vi "Iniciar.vi"() -> ()   [LabVIEW 2015]
uses:
  <vilib>/addons/_office/excel.llb/Excel Get Data (i32).vi
  <vilib>/Utility/NIReport.llb/NI_report.lvclass
  <vilib>/Utility/NIReport.llb/Excel/NI_Excel.lvclass
  <vilib>/addons/_office/NI_ReportGenerationToolkit.lvlib
panel:
  out "Init Data Out":u16[](array[numeric])
  out "Sheet 3 Data":i32
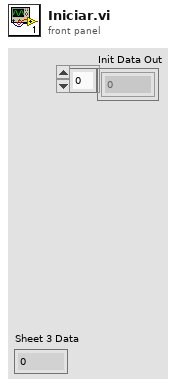
[diagram p1: front panel]
types:
  T1 = enum16{"Standard Report", "HTML", "Word", "Excel"}
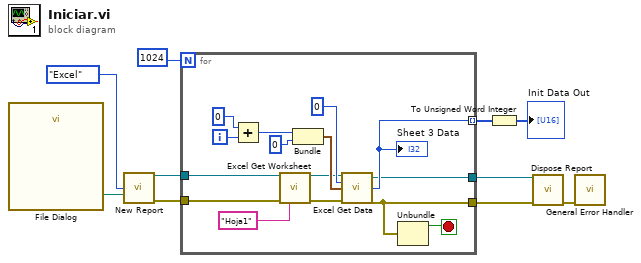
[diagram p0: block diagram]
diagram:
  n1 = call "File Dialog"() -> ("selected path"=w7:path)  [unwired: 7 in, 8 out]
  n2 = call <vilib>:"New Report.vi"("report type"=T1."Excel", "template (empty)"=w7) -> ("report out"=w5:refnum<class "NI_report.lvclass">, "error out"=w4:errorcluster)  [unwired: 4 in, 8 out]
  n3 = for {
    N: 1024 -> [_]
    tunnel: [w16] -> w9 mode=indexing
    tunnel: w5 -> [w15]
    tunnel: w4 -> [w14]
    tunnel: [w13] -> w2
    tunnel: [w12] -> w1
    i -> [w19]
    stop <- w11 stop-if-true
    n4 = Add(x=0, y=w19) -> (x+y=w17:i32)
    n5 = call <vilib>:"Excel Get Worksheet.vi"("report in"=w15, "error in (no error)"=w14, "name (\"\")"="Hoja1" ("name (\"\")")) -> ("report out"=w22:refnum<class "NI_report.lvclass">, "error out"=w21:errorcluster)  [unwired: 1 in, 10 out]
    n6 = Bundle(w17, "worksheet index (0)"=0) -> (w25:cluster{i32, "worksheet index (0)":i32})  [unwired: 1 in]
    n7 = call-poly <vilib>:"Excel Get Data.vi"("report in"=w22, "data type"=0, "start (0, 0)"=w25, "error in (no error)"=w21) -> ("report out"=w13:refnum<class "NI_report.lvclass">, "data"=w16:i32, "error out"=w12:errorcluster)  [unwired: 9 out]
    "Sheet 3 Data" <- w16
    n8 = Unbundle(w12) -> ("status"=w11:bool)  [unwired: 2 out]
  }
  n9 = To Unsigned Word Integer(number=w9) -> (unsigned 16bit integer=→"Init Data Out":u16[])
  n10 = call-dynamic "Dispose Report.vi"("report in"=w2, "error in (no error)"=w1) -> ("error out"=w3:errorcluster)  [unwired: 3 in, 10 out]
  n11 = call <vilib>:"General Error Handler.vi"("error in (no error)"=w3) -> ()  [unwired: 3 in, 12 out]
